vi "Zero N LSBs.vi"(0 "input":u32, 7 "N":i32, 11 "error in (no error)":errorcluster) -> (4 "quantized output":u32, 15 "error out":errorcluster)   [LabVIEW 2017, in "NI_FpgaMspHost.lvlib"]
uses:
  <vilib>/rvi/Analysis/host/Public/NI_FpgaMspHost.lvlib
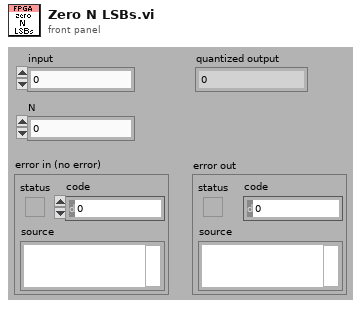
[diagram p1: front panel]
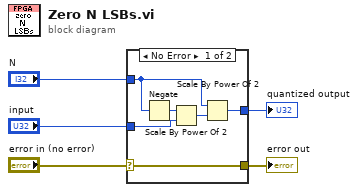
[diagram p0: block diagram]
diagram:
  n1 = case shown="No Error" "error in (no error)" {
    selector: "error in (no error)" -> [w6 w13]
    tunnel: "N" -> [w10 _]
    tunnel: "input" -> [w8 w12]
    tunnel: [w7 w12] -> w3
    tunnel: [w6 w13] -> w1
    frame No Error {
      n2 = Negate(x=w10) -> (-x=w11:i32)
      n3 = Scale By Power Of 2(n=w11, x=w8) -> (x*2^n=w9:u32)
      n4 = Scale By Power Of 2(n=w10, x=w9) -> (x*2^n=w7:u32)
    }
    frame Error {
    }
  }
  "quantized output" <- w3
  "error out" <- w1
